vi "ProcessName.vi"() -> (1 "ProcessName":string)   [LabVIEW 2017, in "TracePointSynchronizer.lvlib"]
uses:
  <vilib>/addons/InsightCM/Devices/Shared/Common/TracePointSynchronizer/TracePointSynchronizer.lvlib
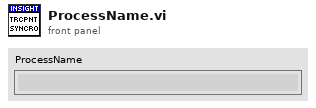
[diagram p1: front panel]
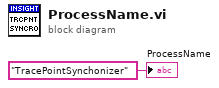
[diagram p0: block diagram]
diagram:
  "ProcessName" <- "TracePointSynchonizer" ("ProcessName")
